vi "Close.vi"(11 "ScopeBase in":refnum<class "ScopeBase.lvclass">) -> (0 "error out":errorcluster)   [LabVIEW 2018, in "ScopeBase.lvclass"]
uses:
  ScopeBase.lvclass
  ScopeBase.lvclass/ScopeBase.ctl
  FpgaRef/FpgaRefBase/FpgaRefBase.lvclass
  Communication/Driver/RemoteConnection/RemoteConnection.lvclass
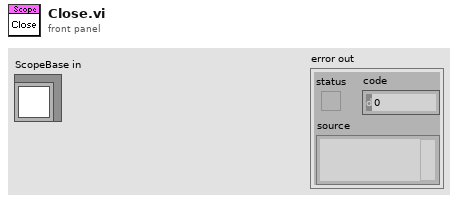
[diagram p1: front panel]
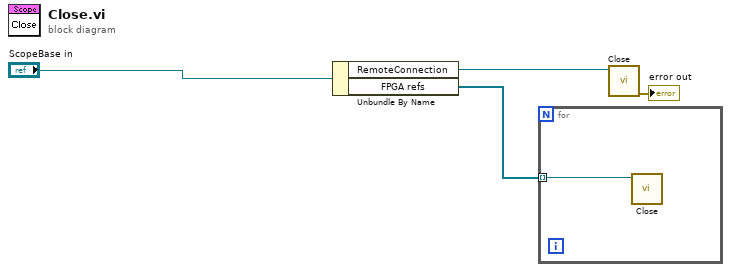
[diagram p0: block diagram]
diagram:
  n1 = Unbundle By Name("ScopeBase in") -> ("RemoteConnection"=w3:refnum<class "RemoteConnection.lvclass">, "FPGA refs"=w2:refnum<class "FpgaRefBase.lvclass">[])
  n2 = for {
    tunnel: w2 -> [w5] mode=indexing
    n3 = call-dynamic "Close.vi"("FpgaRefBase In"=w5) -> ()  [unwired: 11 in]
  }
  n4 = call "Close.vi"("RemoteConnection in"=w3) -> ("error out"=→"error out":errorcluster)  [unwired: 9 in, 1 out]
